vi "Interpolation test.vi"() -> ()   [LabVIEW 2014]
uses:
  <vilib>/rvi/interface/RandomDataEmulation/nirviRandomDataOpen.vi
  <vilib>/rvi/interface/common/niFpgaCacheSessionInfoDynamic.vi
  <vilib>/rvi/interface/common/niFpgaWaitOnOcc.vi
  <vilib>/Utility/error.llb/Error Cluster From Error Code.vi
  <vilib>/rvi/errors/niLvFpgaAdjustHostInterfaceError.vi
  <vilib>/Utility/file.llb/Write To Spreadsheet File (DBL).vi
  <vilib>/FPGAPlugInAG/Dynamic/niLvFpga_Close_Dynamic.vi
  <vilib>/rvi/interface/nirviOpenFPGA/nirviOpenFPGA.xnode
  FPGA Target/Test VIs/FFT Simulation test.vi
  <vilib>/rvi/interface/nirviMethod/nirviMethod.xnode
  <vilib>/rvi/interface/nirviCloseFPGA/nirviCloseFPGA.xnode
  <vilib>/FPGAPlugInAG/Dynamic/niLvFpga_ConfigureFifo_Dynamic.vi
  <vilib>/rvi/errors/niLvFpgaMergeErrorWithErrorCode.vi
  <vilib>/FPGAPlugInAG/Dynamic/niLvFpga_StartFifo_Dynamic.vi
  <vilib>/FPGAPlugInAG/Dynamic/niLvFpga_ReadFifo_Dynamic.vi
  <vilib>/rvi/Analysis/host/Public/NI_FpgaMspHost.lvlib
panel:
  out "McLeod Error":dbl
  out "McLeod":dbl
  out "Theoretical Freq.":dbl
  out "Quinn 2 error":dbl
  out "Quinn 1 error":dbl
  out "Barycentric error":dbl
  out "Quadratic error":dbl
  out "Jain error":dbl
  out "Quinn 2":dbl
  out "Quinn 1":dbl
  out "Barycentric":dbl
  out "Quadratic":dbl
  out "jain":dbl
  in  "#iteration":i32=1
  in  "#Periods":dbl=100.0
  in  "Gen. Freq.":dbl=50000000.0 format="%#_13g"
  in  "#Samples":dbl=1250.0
  in  "Sample Rate (S/s)":dbl=50000000.0 format="%#_13g"
  out "Waveform Graph":dbl[](graph)
  out "Signal":waveform(dbl)(graph)
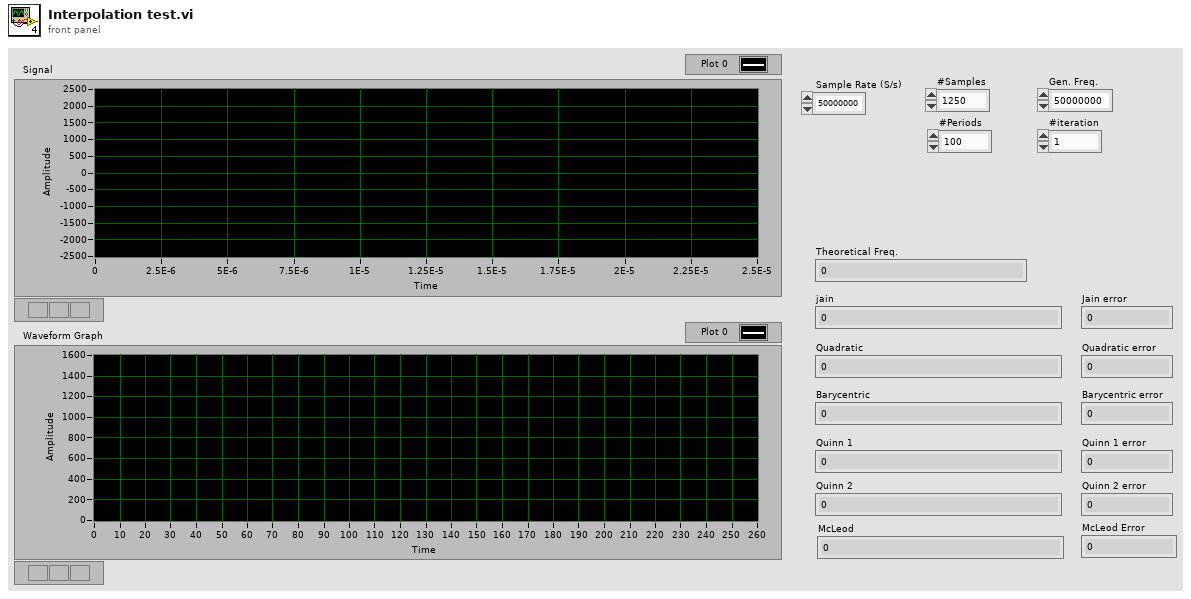
[diagram p1: front panel]
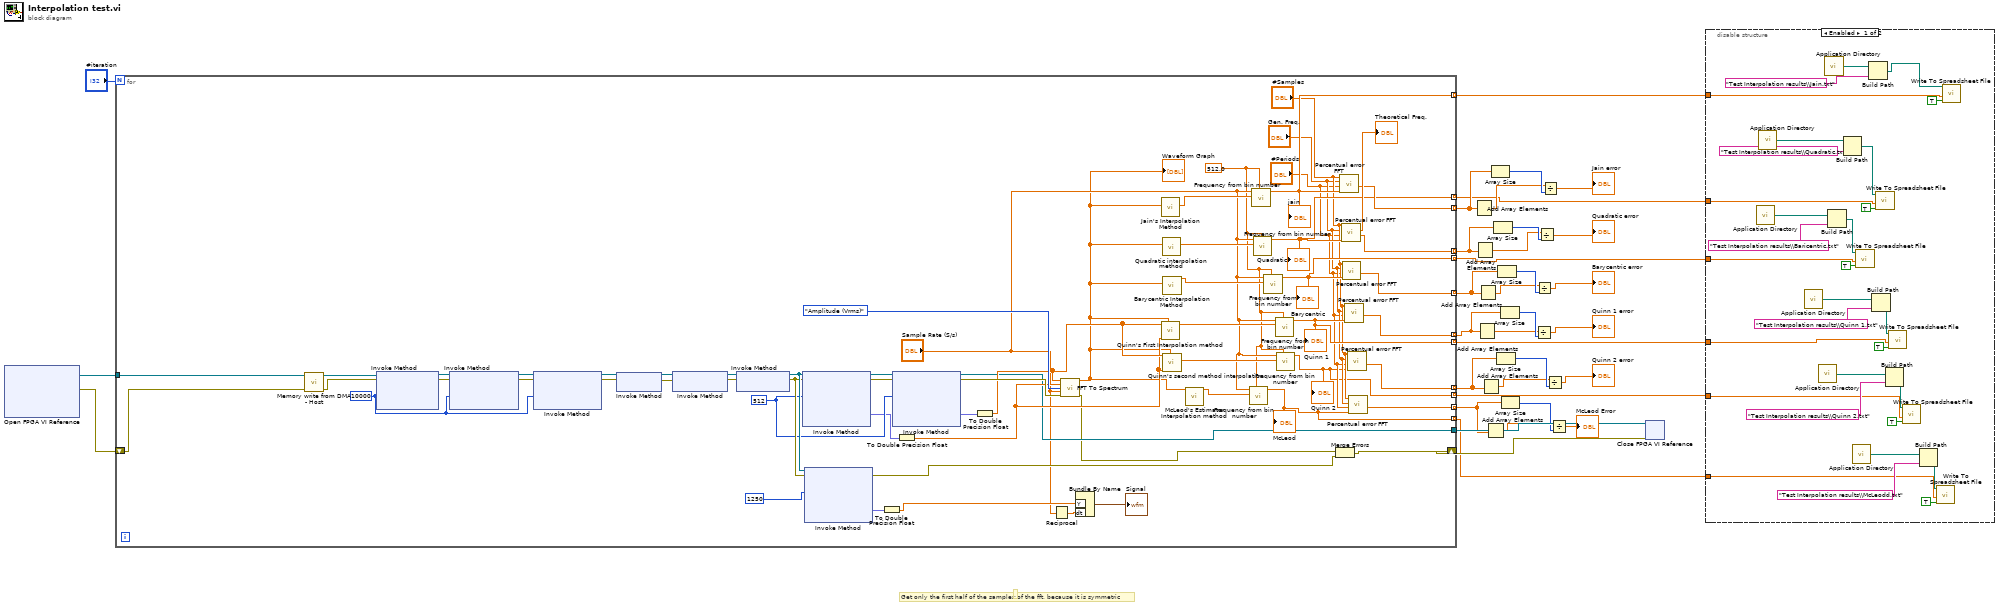
[diagram p0: block diagram]
diagram:
  # "."
  # "Get only the first half of the samples of the fft, because it is symmetric"
  n1 = xnode "Open FPGA VI Reference"() -> ("FPGA VI Reference Out"=w34:refnum<k20>, "error out"=w32:errorcluster)  [unwired: 2 in]
  n2 = for {
    N: "#iteration" -> [_]
    tunnel: w34 -> [w60]
    tunnel: [w59] -> w33
    shift-right: [w55] -> w31
    shift-left: w32 -> [w58]
    tunnel: [w54] -> w12 mode=indexing
    tunnel: [w53] -> w11 mode=indexing
    tunnel: [w52] -> w30 mode=indexing
    tunnel: [w51] -> w13 mode=indexing
    tunnel: [w50] -> w14 mode=indexing
    tunnel: [w49] -> w10 mode=indexing
    tunnel: [w48] -> w9 mode=indexing
    tunnel: [w47] -> w8 mode=indexing
    tunnel: [w46] -> w7 mode=indexing
    tunnel: [w39] -> w4 mode=indexing
    tunnel: [w38] -> w2 mode=indexing
    tunnel: [w37] -> w1 mode=indexing
    w43 = 512.0 ("FFT size")
    w80 = u32 512 ("Requested Depth")
    w93 = u32 10000 ("Requested Depth")
    n3 = call "Memory write from DMA - Host.vi"("error in"=w58, "FPGA VI Reference In"=w60) -> ("error out"=w69:errorcluster, "FPGA VI Reference Out"=w70:refnum<k20>)  [unwired: 6 in, 2 out]
    n4 = xnode "Invoke Method"("FPGA VI Reference In"=w70, "error in"=w69, "Requested Depth"=w93) -> ("FPGA VI Reference Out"=w95:refnum<k20>, "error out"=w94:errorcluster)  [unwired: 1 out]
    n5 = xnode "Invoke Method"("FPGA VI Reference In"=w95, "error in"=w94, "Requested Depth"=w93) -> ("FPGA VI Reference Out"=w92:refnum<k20>, "error out"=w91:errorcluster)  [unwired: 1 out]
    n6 = xnode "Invoke Method"("FPGA VI Reference In"=w92, "error in"=w91, "Requested Depth"=w93) -> ("FPGA VI Reference Out"=w90:refnum<k20>, "error out"=w89:errorcluster)  [unwired: 1 out]
    n7 = xnode "Invoke Method"("FPGA VI Reference In"=w90, "error in"=w89) -> ("FPGA VI Reference Out"=w88:refnum<k20>, "error out"=w87:errorcluster)
    n8 = xnode "Invoke Method"("FPGA VI Reference In"=w88, "error in"=w87) -> ("FPGA VI Reference Out"=w83:refnum<k20>, "error out"=w86:errorcluster)
    n9 = xnode "Invoke Method"("FPGA VI Reference In"=w83, "error in"=w86) -> ("FPGA VI Reference Out"=w82:refnum<k20>, "error out"=w81:errorcluster)
    n10 = xnode "Invoke Method"("FPGA VI Reference In"=w82, "error in"=w81, "Number of Elements"=w80) -> ("FPGA VI Reference Out"=w85:refnum<k20>, "error out"=w84:errorcluster, "Data"=w73:fxp<+/-,22,22>[])  [unwired: 1 in, 1 out]
    n11 = xnode "Invoke Method"("FPGA VI Reference In"=w82, "error in"=w81, "Number of Elements"=u32 1250) -> ("error out"=w56:errorcluster, "Data"=w79:fxp<+/-,12,12>[])  [unwired: 1 in, 2 out]
    n12 = To Double Precision Float(number=w79) -> (double precision float=w77:dbl[])
    n13 = xnode "Invoke Method"("FPGA VI Reference In"=w85, "error in"=w84, "Number of Elements"=w80) -> ("FPGA VI Reference Out"=w59:refnum<k20>, "error out"=w75:errorcluster, "Data"=w74:fxp<+/-,22,22>[])  [unwired: 1 in, 1 out]
    n14 = To Double Precision Float(number=w73) -> (double precision float=w67:dbl[])
    n15 = To Double Precision Float(number=w74) -> (double precision float=w68:dbl[])
    n16 = Reciprocal(x="Sample Rate (S/s)") -> (1/x=w76:dbl)
    n17 = call <vilib>:"FFT To Spectrum.vi"("real FFT data"=w68, "imaginary FFT data"=w67, "spectrum type"=enum8{"Power (Vrms^2)", "Amplitude (Vrms)"}."Amplitude (Vrms)", "sample rate (S/s)"="Sample Rate (S/s)", "error in (no error)"=w75) -> ("spectrum out"=w36:dbl[], "error out"=w57:errorcluster)  [unwired: 8 in, 1 out]
    "Waveform Graph" <- w36
    n18 = Bundle By Name("Y"=w77, "dt"=w76) -> (→"Signal":waveform(dbl))  [unwired: 1 in]
    n19 = call "Jain's Interpolation Method.vi"("FFT array"=w36) -> ("Index Bin"=w66:dbl)  [unwired: 9 in, 1 out]
    n20 = call "Quinn's First Interpolation method.vi"("FFT  spectrum"=w36, "FFT array Im"=w67, "FFT array Re"=w68) -> ("Index Bin"=w64:dbl)  [unwired: 7 in, 1 out]
    n21 = call "Quadratic interpolation method.vi"("FFT array"=w36) -> ("Index Bin"=w62:dbl)  [unwired: 10 in]
    n22 = call "Barycentric Interpolation Method.vi"("FFT array"=w36) -> ("Index Bin"=w63:dbl)  [unwired: 9 in, 1 out]
    n23 = call "Quinn's second method interpolation.vi"("FFT spectrum"=w36, "FFT Imm"=w67, "FFT real"=w68) -> ("Index Bin"=w65:dbl)  [unwired: 8 in]
    n24 = call "McLeod's Estimator Interpolation method.vi"("FFT array"=w36) -> ("Index Bin"=w45:dbl)  [unwired: 9 in, 1 out]
    n25 = call "Frequency from bin number.vi"("FFT size"=w43, "Bin number"=w45, "Sample Rate (S/s)"="Sample Rate (S/s)") -> ("Detected Frequency (Hz)"=w37:dbl)  [unwired: 8 in]
    "McLeod" <- w37
    n26 = call "Frequency from bin number.vi"("FFT size"=w43, "Bin number"=w66, "Sample Rate (S/s)"="Sample Rate (S/s)") -> ("Detected Frequency (Hz)"=w49:dbl)  [unwired: 8 in]
    "jain" <- w49
    n27 = call "Frequency from bin number.vi"("FFT size"=w43, "Bin number"=w62, "Sample Rate (S/s)"="Sample Rate (S/s)") -> ("Detected Frequency (Hz)"=w48:dbl)  [unwired: 8 in]
    "Quadratic" <- w48
    n28 = call "Frequency from bin number.vi"("FFT size"=w43, "Bin number"=w63, "Sample Rate (S/s)"="Sample Rate (S/s)") -> ("Detected Frequency (Hz)"=w47:dbl)  [unwired: 8 in]
    "Barycentric" <- w47
    n29 = call "Frequency from bin number.vi"("FFT size"=w43, "Bin number"=w64, "Sample Rate (S/s)"="Sample Rate (S/s)") -> ("Detected Frequency (Hz)"=w46:dbl)  [unwired: 8 in]
    "Quinn 1" <- w46
    n30 = call "Frequency from bin number.vi"("FFT size"=w43, "Bin number"=w65, "Sample Rate (S/s)"="Sample Rate (S/s)") -> ("Detected Frequency (Hz)"=w38:dbl)  [unwired: 8 in]
    "Quinn 2" <- w38
    n31 = Merge Errors(w57, w56) -> (w55:errorcluster)
    n32 = call "Percentual error FFT.vi"("Detected Freq"=w49, "#Periods"="#Periods", "Gen. Freq."="Gen. Freq.", "#Samples"="#Samples") -> ("Error %"=w50:dbl)  [unwired: 6 in, 1 out]
    n33 = call "Percentual error FFT.vi"("Detected Freq"=w48, "#Periods"="#Periods", "Gen. Freq."="Gen. Freq.", "#Samples"="#Samples") -> ("Error %"=w51:dbl, "Theoretical Freq."=→"Theoretical Freq.":dbl)  [unwired: 6 in]
    n34 = call "Percentual error FFT.vi"("Detected Freq"=w47, "#Periods"="#Periods", "Gen. Freq."="Gen. Freq.", "#Samples"="#Samples") -> ("Error %"=w54:dbl)  [unwired: 6 in, 1 out]
    n35 = call "Percentual error FFT.vi"("Detected Freq"=w46, "#Periods"="#Periods", "Gen. Freq."="Gen. Freq.", "#Samples"="#Samples") -> ("Error %"=w53:dbl)  [unwired: 6 in, 1 out]
    n36 = call "Percentual error FFT.vi"("Detected Freq"=w38, "#Periods"="#Periods", "Gen. Freq."="Gen. Freq.", "#Samples"="#Samples") -> ("Error %"=w52:dbl)  [unwired: 6 in, 1 out]
    n37 = call "Percentual error FFT.vi"("Detected Freq"=w37, "#Periods"="#Periods", "Gen. Freq."="Gen. Freq.", "#Samples"="#Samples") -> ("Error %"=w39:dbl)  [unwired: 6 in, 1 out]
  }
  n38 = Add Array Elements(numeric array=w14) -> (sum=w28:dbl)
  n39 = Add Array Elements(numeric array=w13) -> (sum=w26:dbl)
  n40 = Add Array Elements(numeric array=w11) -> (sum=w22:dbl)
  n41 = Add Array Elements(numeric array=w12) -> (sum=w24:dbl)
  n42 = Add Array Elements(numeric array=w30) -> (sum=w20:dbl)
  n43 = Add Array Elements(numeric array=w4) -> (sum=w6:dbl)
  n44 = Array Size(array=w14) -> (size(s)=w29:i32)
  n45 = Array Size(array=w13) -> (size(s)=w27:i32)
  n46 = Array Size(array=w30) -> (size(s)=w21:i32)
  n47 = Array Size(array=w12) -> (size(s)=w25:i32)
  n48 = Array Size(array=w11) -> (size(s)=w23:i32)
  n49 = Array Size(array=w4) -> (size(s)=w5:i32)
  n50 = Divide(x=w22, y=w23) -> (x/y=→"Quinn 1 error":dbl)
  n51 = Divide(x=w24, y=w25) -> (x/y=→"Barycentric error":dbl)
  n52 = Divide(x=w26, y=w27) -> (x/y=→"Quadratic error":dbl)
  n53 = Divide(x=w28, y=w29) -> (x/y=→"Jain error":dbl)
  n54 = Divide(x=w20, y=w21) -> (x/y=→"Quinn 2 error":dbl)
  n55 = Divide(x=w6, y=w5) -> (x/y=→"McLeod Error":dbl)
  n56 = xnode "Close FPGA VI Reference"("FPGA VI Reference In"=w33, "error in"=w31) -> ()  [unwired: 1 out]
  n57 = disable-structure shown="Enabled" {
    disable-tunnel: w10 -> [w121 _]
    disable-tunnel: w9 -> [w120 _]
    disable-tunnel: w8 -> [w119 _]
    disable-tunnel: w7 -> [w118 _]
    disable-tunnel: w2 -> [w102 _]
    disable-tunnel: w1 -> [w98 _]
    frame Enabled {
      n58 = call <vilib>:"Application Directory.vi"() -> ("Application Directory"=w115:path)
      n59 = call <vilib>:"Application Directory.vi"() -> ("Application Directory"=w114:path)
      n60 = call <vilib>:"Application Directory.vi"() -> ("Application Directory"=w117:path)
      n61 = call <vilib>:"Application Directory.vi"() -> ("Application Directory"=w105:path)
      n62 = call <vilib>:"Application Directory.vi"() -> ("Application Directory"=w108:path)
      n63 = Build Path(base path=w115, name or relative path="Test Interpolation results\\Baricentric.txt") -> (appended path=w112:path)
      n64 = Build Path(base path=w114, name or relative path="Test Interpolation results\\Quadratic.txt") -> (appended path=w113:path)
      n65 = call <vilib>:"Application Directory.vi"() -> ("Application Directory"=w101:path)
      n66 = call-poly <vilib>:"Write To Spreadsheet File.vi"("append to file? (new file:F)"=TRUE, "1D data"=w119, "file path (dialog if empty)"=w112) -> ()  [unwired: 5 in, 1 out]
      n67 = Build Path(base path=w108, name or relative path="Test Interpolation results\\Jain.txt") -> (appended path=w106:path)
      n68 = Build Path(base path=w117, name or relative path="Test Interpolation results\\Quinn 1.txt") -> (appended path=w116:path)
      n69 = call-poly <vilib>:"Write To Spreadsheet File.vi"("append to file? (new file:F)"=TRUE, "1D data"=w120, "file path (dialog if empty)"=w113) -> ()  [unwired: 5 in, 1 out]
      n70 = Build Path(base path=w105, name or relative path="Test Interpolation results\\Quinn 2.txt") -> (appended path=w104:path)
      n71 = call-poly <vilib>:"Write To Spreadsheet File.vi"("append to file? (new file:F)"=TRUE, "1D data"=w118, "file path (dialog if empty)"=w116) -> ()  [unwired: 5 in, 1 out]
      n72 = call-poly <vilib>:"Write To Spreadsheet File.vi"("append to file? (new file:F)"=TRUE, "1D data"=w102, "file path (dialog if empty)"=w104) -> ()  [unwired: 5 in, 1 out]
      n73 = Build Path(base path=w101, name or relative path="Test Interpolation results\\McLeodd.txt") -> (appended path=w100:path)
      n74 = call-poly <vilib>:"Write To Spreadsheet File.vi"("append to file? (new file:F)"=TRUE, "1D data"=w98, "file path (dialog if empty)"=w100) -> ()  [unwired: 5 in, 1 out]
      n75 = call-poly <vilib>:"Write To Spreadsheet File.vi"("append to file? (new file:F)"=TRUE, "1D data"=w121, "file path (dialog if empty)"=w106) -> ()  [unwired: 5 in, 1 out]
    }
    frame Disabled {
    }
  }
